vi "Get Ctrl Info.vi"(8 "error in (no error)":errorcluster, 9 "GObj Refnum":refnum<vi>, 10 "VI-Ref":refnum<vi>, 11 "Ctrl Reference's in":refnum<class "Ctrl Reference's.lvclass">) -> (0 "error out":errorcluster, 1 "Has Label?":bool, 2 "Label":string, 3 "Ctrl Reference's out":refnum<class "Ctrl Reference's.lvclass">)   [LabVIEW 2023, in "Ctrl Reference's.lvclass"]
uses:
  Ctrl Reference's.lvclass
  Ctrl Reference's.lvclass/Ctrl Reference's.ctl
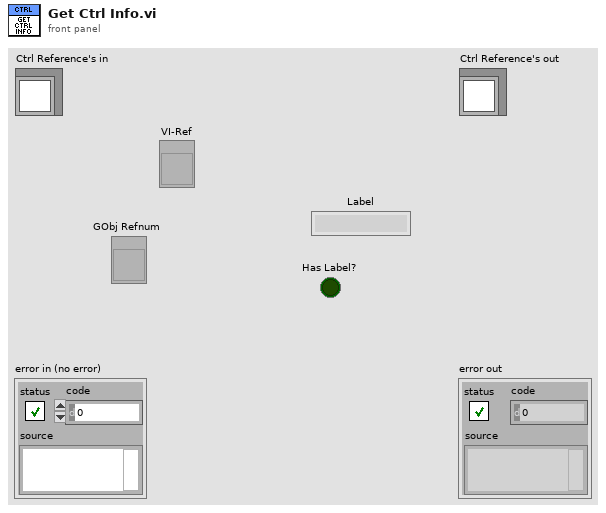
[diagram p1: front panel]
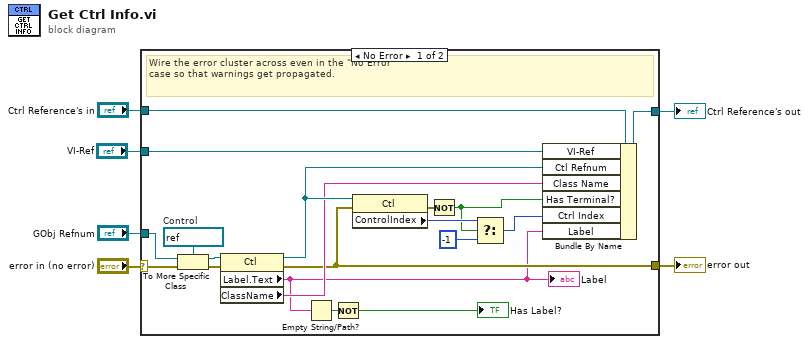
[diagram p0: block diagram]
diagram:
  n1 = case shown="No Error" "error in (no error)" {
    selector: "error in (no error)" -> [w16 w27]
    tunnel: [w10 w27] -> w5
    tunnel: [w24 w26] -> w3
    tunnel: "Ctrl Reference's in" -> [w25 w26]
    tunnel: "GObj Refnum" -> [w15 _]
    tunnel: "VI-Ref" -> [w8 _]
    frame No Error {
      w23 = refnum<vi> refnum  # Control
      # "Wire the error cluster across even in the \"No Error\"\ncase so that warnings get propagated."
      n2 = To More Specific Class(target class=w23, reference=w15, error in=w16) -> (specific class reference=w22:refnum<vi>, error out=w21:errorcluster)
      n3 = property class="Ctl"(reference=w22, error in=w21) -> (reference out=w14:refnum<vi>, error out=w10:errorcluster, "Label.Text"=w7:string, "ClassName"=w13:string)
      "Label" <- w7
      n4 = Empty String/Path?(string/path=w7) -> (empty?=w20:bool)
      n5 = Not(x=w20) -> (.not. x?=→"Has Label?":bool)
      n6 = property class="Ctl"(reference=w14, error in=w10) -> (error out=w19:errorcluster, "ControlIndex"=w18:i32)  [unwired: 1 out]
      n7 = Not(x=w19) -> (.not. x?=w12:bool)
      n8 = Select(t=w18, s=w12, f=-1) -> (s? t:f=w11:i32)
      n9 = Bundle By Name(cluster=w25, "VI-Ref"=w8, "Ctl Refnum"=w14, "Class Name"=w13, "Has Terminal?"=w12, "Ctrl Index"=w11, "Label"=w7) -> (w24:refnum<class "Ctrl Reference's.lvclass">)
    }
    frame Error {
    }
  }
  "error out" <- w5
  "Ctrl Reference's out" <- w3
